vi "w_bridge_calc.vi"(0 "R1":dbl, 1 "R2":dbl, 2 "Ei":dbl, 3 "R3":dbl, 4 "R4":dbl) -> (5 "Eo":dbl, 6 "R2 (if unknown)":dbl)   [LabVIEW 2019]
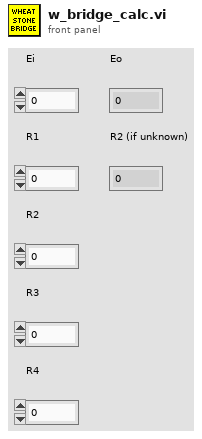
[diagram p1: front panel]
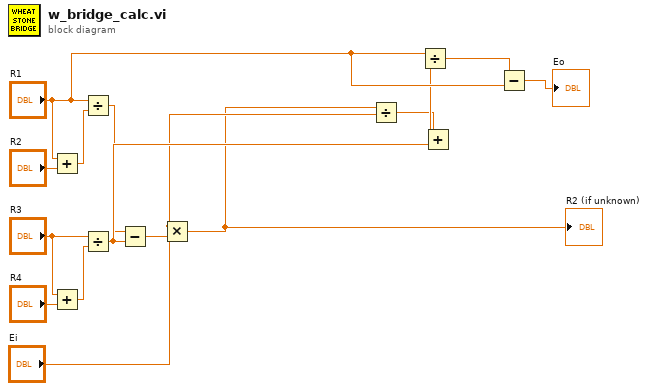
[diagram p0: block diagram]
diagram:
  n1 = Add(x="R1", y="R2") -> (x+y=w2:dbl)
  n2 = Add(x="R3", y="R4") -> (x+y=w4:dbl)
  n3 = Divide(x="R1", y=w2) -> (x/y=w3:dbl)
  n4 = Divide(x="R3", y=w4) -> (x/y=w10:dbl)
  n5 = Subtract(x=w3, y=w10) -> (x-y=w7:dbl)
  n6 = Multiply(x="Ei", y=w7) -> (x*y=w8:dbl)
  "R2 (if unknown)" <- w8
  n7 = Divide(x=w8, y="Ei") -> (x/y=w11:dbl)
  n8 = Add(x=w11, y=w10) -> (x+y=w12:dbl)
  n9 = Divide(x="R1", y=w12) -> (x/y=w14:dbl)
  n10 = Subtract(x=w14, y="R1") -> (x-y=→"Eo":dbl)
